vi "Entity Definition OoC.vi"(11 "Entity path":path) -> (0 "error out":errorcluster, 3 "Definition":refnum<class "Type.lvclass">[](array[class]), 5 "Result Types":string[](array[string]))   [LabVIEW 2020, in "Conditum-Tools.lvlib" / "Entity Editor.lvclass"]
uses:
  Entity Editor.lvclass
  Conditum-Clone/Columns/Type/Type.lvclass
  <vilib>/IlluminatedG/IG Conditum Base/Conditum/Entity/Entity.lvclass
  88afa94e-ab6a-4518-8d0d-0b7e4e3fb94a.vi
  <vilib>/Utility/LVClass/Get LV Class Name.vi
  <vilib>/Utility/error.llb/Error Cluster From Error Code.vi
  Conditum-Tools.lvlib
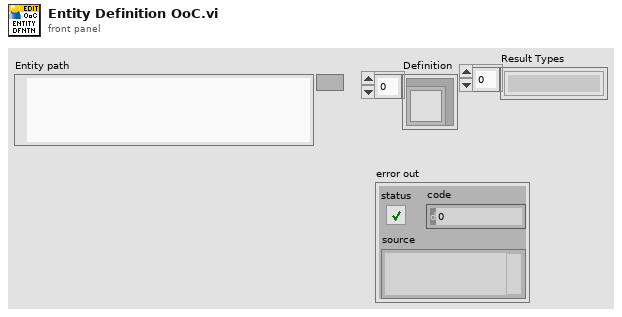
[diagram p1: front panel]
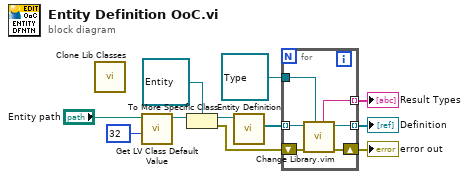
[diagram p0: block diagram]
diagram:
  n1 = call "Clone Lib Classes.vi"() -> ()  [unwired: 12 in]
  n2 = call <vilib>:"Get LV Class Default Value.vi"("options"=u32 32, "class path"="Entity path") -> ("object"=w11:refnum<class>)  [unwired: 8 in, 1 out]
  n3 = To More Specific Class(target class=refnum<class "Entity.lvclass"> refnum ("Conditum:Entity"), reference=w11) -> (specific class reference=w4:refnum<class "Entity.lvclass">, error out=w2:errorcluster)  [unwired: 1 in]
  n4 = call <vilib>:"Entity Definition.vi"("Entity in"=w4) -> ("Definition"=w3:refnum<class "Type.lvclass">[])  [unwired: 10 in]
  n5 = for {
    tunnel: w3 -> [w17] mode=indexing
    tunnel: refnum<class "Type.lvclass"> refnum ("Conditum:Columns:Type.lvclass") -> [w16]
    tunnel: [w15] -> w5 mode=indexing
    shift-right: [w14] -> w6
    shift-left: w2 -> [w13]
    tunnel: [w12] -> w1 mode=indexing
    n6 = call "Change Library.vim"("To Type"=w16, "error in (no error)"=w13, "From Value"=w17) -> ("error out"=w14:errorcluster, "To Value"=w15:refnum<class "Type.lvclass">, "result string"=w12:string)  [unwired: 6 in]
  }
  "error out" <- w6
  "Definition" <- w5
  "Result Types" <- w1
